vi "DataPacker_ReadThisHostname.vi"(8 "error in (no error)":errorcluster, 11 "DataPacker in":refnum<class "DataPacker.lvclass">) -> (0 "error out":errorcluster, 2 "This Hostname":string, 3 "DataPacker out":refnum<class "DataPacker.lvclass">)   [LabVIEW 2018, in "feGEM DataPacker.lvlib" / "DataPacker.lvclass"]
uses:
  DataPacker.lvclass
  DataPacker.lvclass/DataPacker.ctl
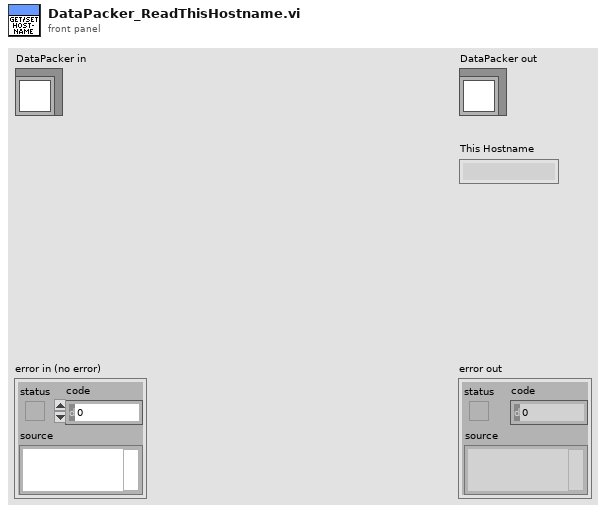
[diagram p1: front panel]
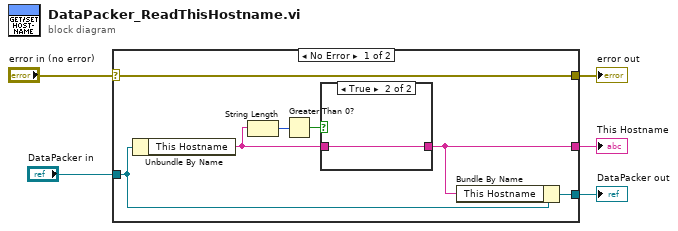
[diagram p0: block diagram]
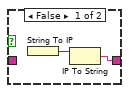
[diagram p2: hidden frame]
diagram:
  n1 = case shown="No Error" "error in (no error)" {
    selector: "error in (no error)" -> [w12 w16]
    tunnel: [w12 w16] -> w4
    tunnel: [w7 w17] -> w2
    tunnel: "DataPacker in" -> [w8 w17]
    tunnel: [w6 _] -> w1
    frame No Error {
      n2 = Unbundle By Name(w8) -> ("This Hostname"=w9:string)
      n3 = String Length(string=w9) -> (length=w11:i32)
      n4 = Greater Than 0?(x=w11) -> (x > 0?=w10:bool)
      n5 = case shown="True" w10 {
        tunnel: [w13 w15] -> w6
        tunnel: w9 -> [_ w15]
        frame False {
          n6 = String To IP() -> (0:w14:u32)  [unwired: 1 in]
          n7 = IP To String(2:w14) -> (0:w13:string)  [unwired: 1 in]
        }
        frame True {
        }
      }
      n8 = Bundle By Name(cluster=w8, "This Hostname"=w6) -> (w7:refnum<class "DataPacker.lvclass">)
    }
    frame Error {
    }
  }
  "error out" <- w4
  "DataPacker out" <- w2
  "This Hostname" <- w1
